vi "transmitModbus.vi"(8 "error in (no error)":errorcluster, 11 "Model in":refnum<class "Model.lvclass">) -> (0 "error out":errorcluster, 3 "Model out":refnum<class "Model.lvclass">)   [LabVIEW 2016, in "Model.lvclass"]
uses:
  Model.lvclass
  Model.lvclass/Model.ctl
  Resources/FPGA/FPGA.lvclass
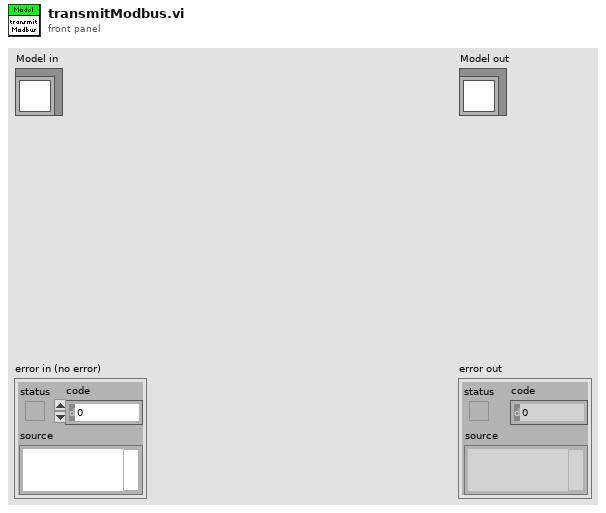
[diagram p1: front panel]
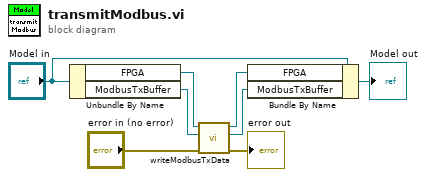
[diagram p0: block diagram]
diagram:
  n1 = Unbundle By Name("Model in") -> ("FPGA"=w6:refnum<class "FPGA.lvclass">, "ModbusTxBuffer"=w5:refnum<class "ModbusBuffer.lvclass">)
  n2 = call "writeModbusTxData.vi"("error in (no error)"="error in (no error)", "ModbusBuffer in"=w5, "FPGA in"=w6) -> ("error out"=→"error out":errorcluster, "ModbusBuffer out"=w2:refnum<class "ModbusBuffer.lvclass">, "FPGA out"=w3:refnum<class "FPGA.lvclass">)  [unwired: 5 in, 1 out]
  n3 = Bundle By Name(cluster="Model in", "FPGA"=w3, "ModbusTxBuffer"=w2) -> (→"Model out":refnum<class "Model.lvclass">)
